vi "AB_Engine_Update_Exe_Timestamp.vi"(8 "error in (no error)":errorcluster, 11 "pathExe":path) -> (0 "error out":errorcluster)   [LabVIEW 2020]
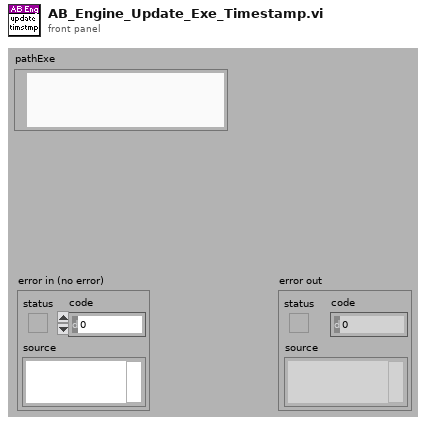
[diagram p1: front panel]
types:
  T1 = enum32{"invalid OS target", "Mac OS", "Windows 3.1", "Windows 95/NT", "Solaris 1", "Solaris 2", "HP-UX", "PowerMAX", "Linux", "Irix", "Rhapsody", "BeOS", "AIX", "OSF1", "VxWorks", "PharLap", "Carbon", "RTX", "Windows x64", "Linux x64", "Mac OS X x64"}
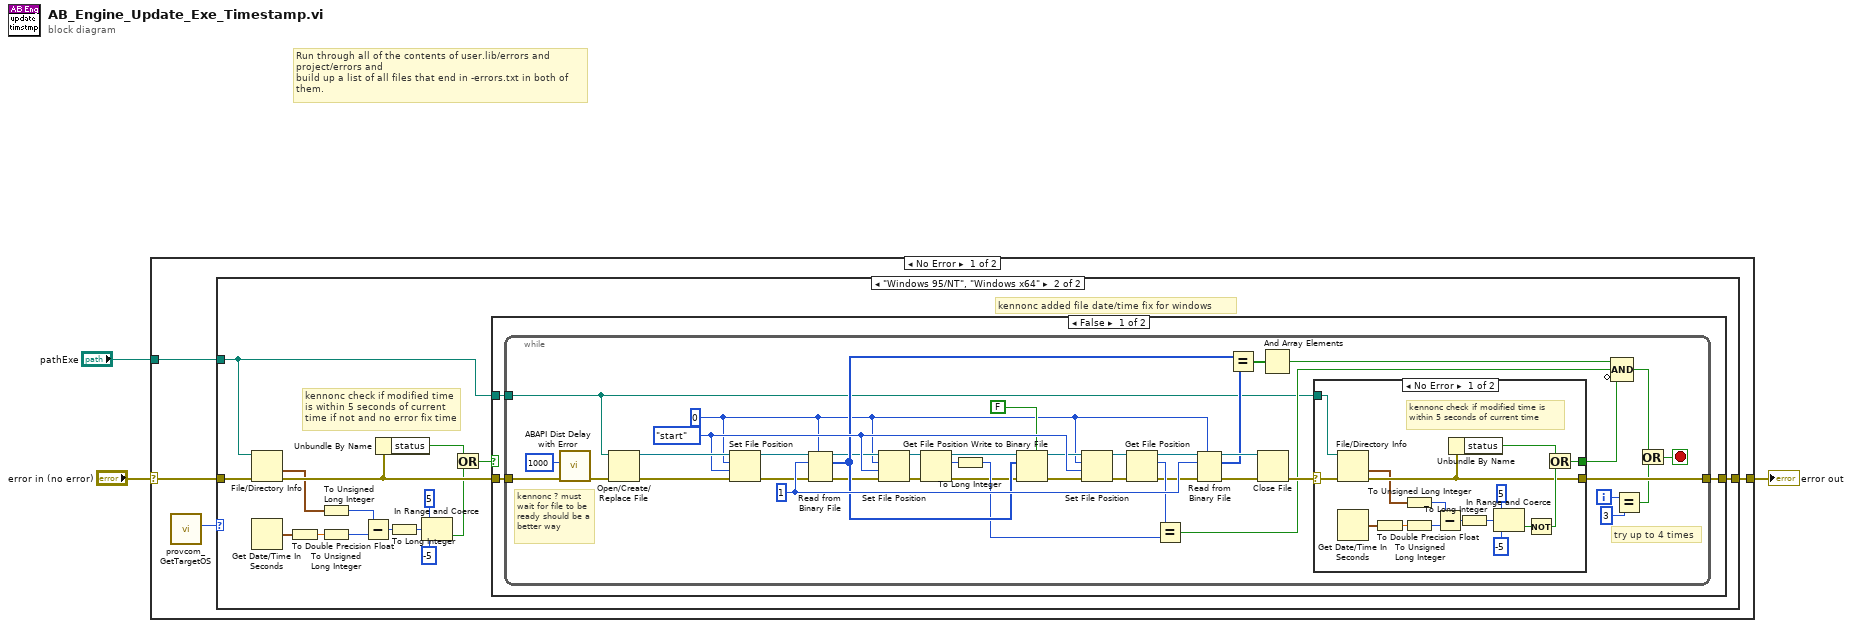
[diagram p0: block diagram]
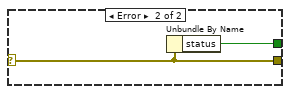
[diagram p3: hidden frame]
diagram:
  # "Run through all of the contents of user.lib/errors and project/errors and\nbuild up a list of all files that end in -errors.txt in both of them."
  n1 = case shown="No Error" "error in (no error)" {
    selector: "error in (no error)" -> [w6 w89]
    tunnel: [w5 w89] -> w2
    tunnel: "pathExe" -> [w7 _]
    frame No Error {
      n2 = call <resource>:"provcom_GetTargetOS.vi"() -> ("App.TargetOS"=w4:T1)  [unwired: 11 in]
      n3 = case shown="\"Windows 95/NT\", \"Windows x64\"" w4 {
        tunnel: [w8 w24] -> w5
        tunnel: w6 -> [w8 w19]
        tunnel: w7 -> [_ w20]
        frame Default {
        }
        frame "Windows 95/NT", "Windows x64" {
          # "kennonc check if modified time is within 5 seconds of current time if not and no error fix time"
          # "kennonc added file date/time fix for windows"
          n4 = File/Directory Info(path=w20, error in=w19) -> (last mod=w9:timestamp, error out=w18:errorcluster)  [unwired: 5 out]
          n5 = Get Date/Time In Seconds() -> (seconds since 1Jan1904=w12:timestamp)
          n6 = To Double Precision Float(number=w12) -> (double precision float=w11:dbl)
          n7 = To Unsigned Long Integer(number=w9) -> (unsigned 32bit integer=w10:u32)
          n8 = To Unsigned Long Integer(number=w11) -> (unsigned 32bit integer=w15:u32)
          n9 = Subtract(x=w10, y=w15) -> (x-y=w21:u32)
          n10 = Unbundle By Name(w18) -> ("status"=w16:bool)
          n11 = To Long Integer(number=w21) -> (32bit integer=w14:i32)
          n12 = In Range and Coerce(upper limit=5 ("x"), x=w14, lower limit=-5 ("x")) -> (In Range?=w13:bool)  [unwired: 1 out]
          n13 = Or(x=w16, y=w13) -> (x .or. y?=w17:bool)
          n14 = case shown="False" w17 {
            tunnel: [w27 w88] -> w24
            tunnel: w18 -> [w25 w88]
            tunnel: w20 -> [w26 _]
            frame False {
              n15 = while {
                tunnel: [w53] -> w27
                tunnel: w26 -> [w50]
                tunnel: w25 -> [w48]
                i -> [w46]
                stop <- w43 stop-if-true
                w60 = 1 ("count")
                w28 = 0 ("pos offset (0)")
                w61 = enum16{"start", "end", "current"}."start" ("pos mode (0:2)")
                # "try up to 4 times"
                # "kennonc ? must wait for file to be ready should be a better way"
                n16 = call <vilib>:"ABAPI Dist Delay with Error.vi"("error in (no error)"=w48, "milliseconds to wait"=u32 1000) -> ("error out"=w49:errorcluster)  [unwired: 9 in]
                n17 = Open/Create/Replace File(file path (use dialog)=w50, error in=w49) -> (refnum out=w69:refnum<file>, error out=w68:errorcluster)  [unwired: 4 in, 1 out]
                n18 = Set File Position(offset (in bytes) (0)=w28, refnum=w69, from (0:start)=w61, error in=w68) -> (refnum out=w33:refnum<file>, error out=w32:errorcluster)
                n19 = Read from Binary File(5:w28, 8:w32, 10:w60, 11:w33) -> (0:w30:errorcluster, 2:w59:i32[], 3:w31:refnum<file>)  [unwired: 2 in, 1 out]
                n20 = Get File Position(4:w30, 7:w31) -> (0:w66:errorcluster, 2:w29:i64, 3:w67:refnum<file>)
                n21 = Set File Position(offset (in bytes) (0)=w28, refnum=w67, from (0:start)=w61, error in=w66) -> (refnum out=w38:refnum<file>, error out=w37:errorcluster)
                n22 = To Long Integer(number=w29) -> (32bit integer=w55:i32)
                n23 = Write to Binary File(file (use dialog)=w38, data=w59, error in=w37, 5:FALSE ("prepend array or string size? (T)")) -> (refnum out=w36:refnum<file>, error out=w35:errorcluster)  [unwired: 2 in, 1 out]
                n24 = Get File Position(4:w35, 7:w36) -> (0:w64:errorcluster, 2:w54:i64, 3:w65:refnum<file>)
                n25 = Set File Position(offset (in bytes) (0)=w28, refnum=w65, from (0:start)=w61, error in=w64) -> (refnum out=w40:refnum<file>, error out=w39:errorcluster)
                n26 = Equal?(x=w54, y=w55) -> (x = y?=w51:bool)
                n27 = Read from Binary File(5:w28, 8:w39, 10:w60, 11:w40) -> (0:w63:errorcluster, 2:w58:i32[], 3:w62:refnum<file>)  [unwired: 2 in, 1 out]
                n28 = Equal?(x=w59, y=w58) -> (x = y?=w57:bool[])
                n29 = Close File(refnum=w62, error in=w63) -> (error out=w56:errorcluster)  [unwired: 1 out]
                n30 = And Array Elements(Boolean array=w57) -> (logical AND=w52:bool)
                n31 = case shown="No Error" w56 {
                  selector: w56 -> [w78 w86]
                  tunnel: [w84 w87] -> w41
                  tunnel: w50 -> [w85 _]
                  tunnel: [w79 w86] -> w53
                  frame No Error {
                    # "kennonc check if modified time is within 5 seconds of current time"
                    n32 = File/Directory Info(path=w85, error in=w78) -> (last mod=w70:timestamp, error out=w79:errorcluster)  [unwired: 5 out]
                    n33 = Get Date/Time In Seconds() -> (seconds since 1Jan1904=w72:timestamp)
                    n34 = To Double Precision Float(number=w72) -> (double precision float=w71:dbl)
                    n35 = To Unsigned Long Integer(number=w70) -> (unsigned 32bit integer=w75:u32)
                    n36 = To Unsigned Long Integer(number=w71) -> (unsigned 32bit integer=w74:u32)
                    n37 = Subtract(x=w75, y=w74) -> (x-y=w83:u32)
                    n38 = Unbundle By Name(w79) -> ("status"=w77:bool)
                    n39 = To Long Integer(number=w83) -> (32bit integer=w73:i32)
                    n40 = In Range and Coerce(upper limit=5 ("x"), x=w73, lower limit=-5 ("x")) -> (In Range?=w76:bool)  [unwired: 1 out]
                    n41 = Not(x=w76) -> (.not. x?=w80:bool)
                    n42 = Or(x=w77, y=w80) -> (x .or. y?=w84:bool)
                  }
                  frame Error {
                    n43 = Unbundle By Name(w86) -> ("status"=w87:bool)
                  }
                }
                n44 = Compound Arithmetic op=AND(w52, w51, invert w41) -> (w42:bool)
                n45 = Equal?(x=w46, y=3) -> (x = y?=w44:bool)
                n46 = Or(x=w42, y=w44) -> (x .or. y?=w43:bool)
              }
            }
            frame True {
            }
          }
        }
      }
    }
    frame Error {
    }
  }
  "error out" <- w2
